vi "9265 AO.vi"() -> ()   [LabVIEW 2020]
uses:
  controls/AO_0_3.ctl
panel:
  out "chiller actuator valve":dbl
  in  "9265 AO":T1
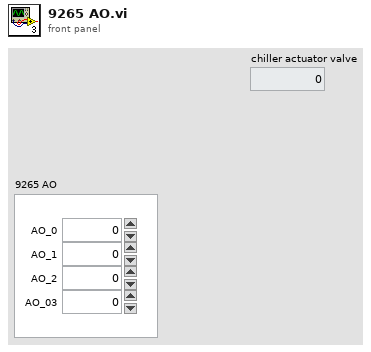
[diagram p1: front panel]
types:
  T1 = typedef "AO_0_3.ctl" = cluster{"AO_0":dbl, "AO_1":dbl, "AO_2":dbl, "AO_03":dbl}
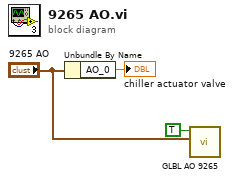
[diagram p0: block diagram]
diagram:
  n1 = Unbundle By Name("9265 AO") -> ("AO_0"=→"chiller actuator valve":dbl)
  n2 = call "GLBL AO 9265.vi"("9265 AO in"="9265 AO", "write_read"=TRUE) -> ()  [unwired: 9 in, 1 out]
